vi "Temp_SetTempOrigin.vi"(8 "Z":dbl format="%#_13g", 9 "Y":dbl format="%#_13g", 10 "X":dbl format="%#_13g", 11 "String":string) -> (3 "concatenated string":string)   [LabVIEW 2016]
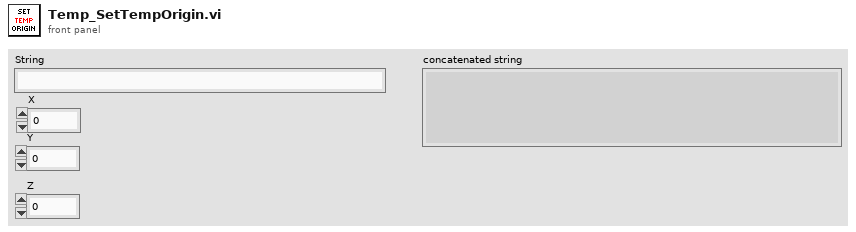
[diagram p1: front panel]
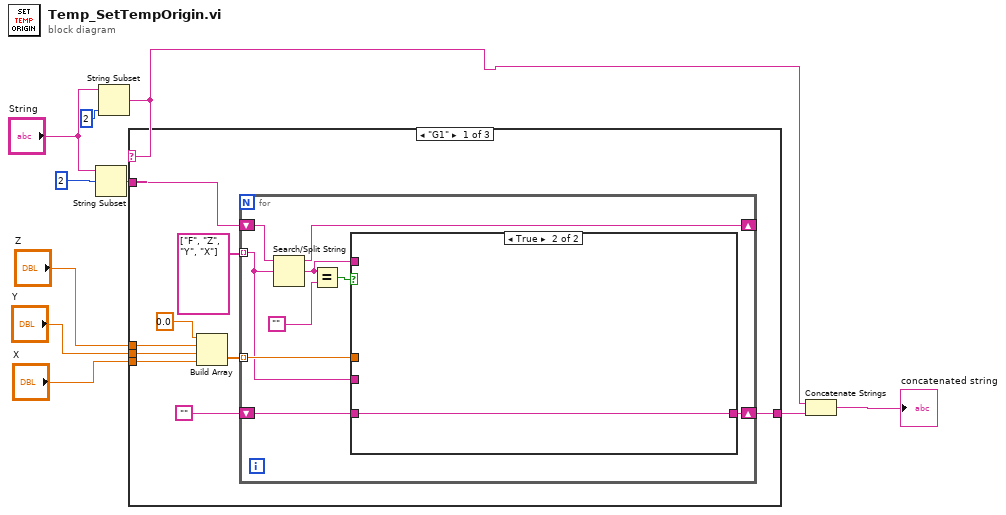
[diagram p0: block diagram]
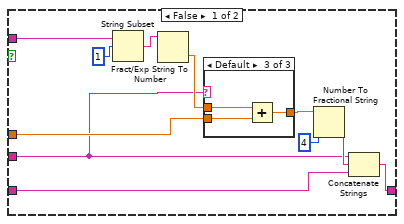
[diagram p2: hidden frame]
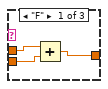
[diagram p3: hidden frame]
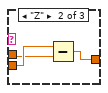
[diagram p4: hidden frame]
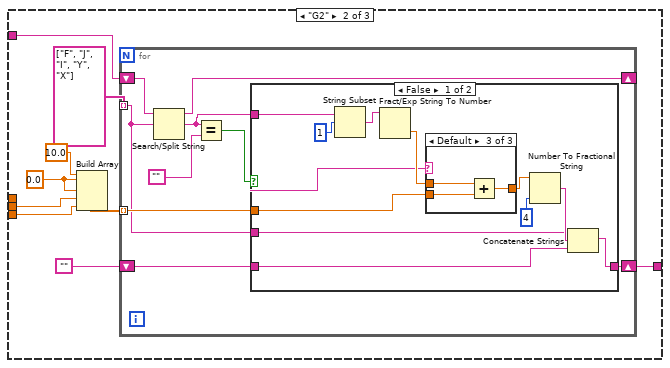
[diagram p5: hidden frame]
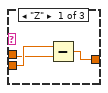
[diagram p6: hidden frame]
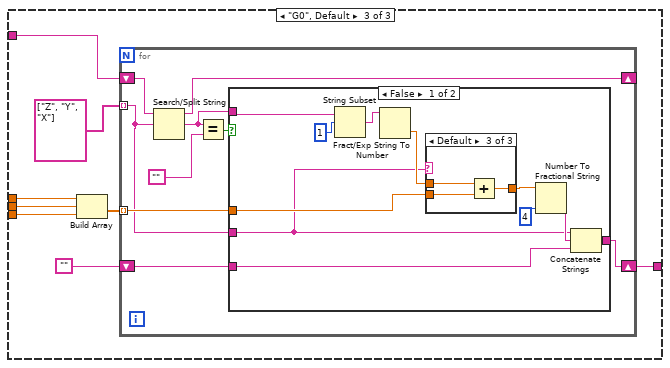
[diagram p9: hidden frame]
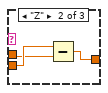
[diagram p11: hidden frame]
diagram:
  n1 = String Subset(string="String", offset (0)=2) -> (substring=w9:string)  [unwired: 1 in]
  n2 = String Subset(string="String", length (rest)=2) -> (substring=w1:string)  [unwired: 1 in]
  n3 = case shown="\"G1\"" w1 {
    tunnel: w9 -> [w18 w57 w94]
    tunnel: "Z" -> [w17 _ w93]
    tunnel: "Y" -> [w16 w51 w92]
    tunnel: "X" -> [w15 w52 w91]
    tunnel: [w11 w54 w88] -> w3
    frame "G1" {
      n4 = Build Array(0.0, w17, w16, w15) -> (w13:dbl[])
      n5 = for {
        tunnel: string[] ["F", "Z", "Y", "X"] -> [w22] mode=indexing
        tunnel: w13 -> [w24] mode=indexing
        shift-right: [w27] -> _
        shift-left: w18 -> [w28]
        shift-right: [w25] -> w11
        shift-left: "" -> [w23]
        n6 = Search/Split String(string=w28, search string/char (-)=w22) -> (substring before match=w27:string, match + rest of string=w20:string)  [unwired: 1 in, 1 out]
        n7 = Equal?(x=w20, y="") -> (x = y?=w21:bool)
        n8 = case shown="True" w21 {
          tunnel: [w34 w49] -> w25
          tunnel: w24 -> [w33 _]
          tunnel: w23 -> [w32 w49]
          tunnel: w22 -> [w31 _]
          tunnel: w20 -> [w29 _]
          frame False {
            n9 = String Subset(string=w29, offset (0)=1) -> (substring=w38:string)  [unwired: 1 in]
            n10 = Fract/Exp String To Number(string=w38) -> (number=w37:dbl)  [unwired: 3 in, 1 out]
            n11 = case shown="Default" w31 {
              tunnel: w37 -> [w41 w43 w48]
              tunnel: [w42 w45 w47] -> w36
              tunnel: w33 -> [w40 w44 w46]
              frame "F" {
                n12 = Add(x=w41, y=w40) -> (x+y=w42:dbl)
              }
              frame "Z" {
                n13 = Subtract(x=w44, y=w43) -> (x-y=w45:dbl)
              }
              frame Default {
                n14 = Add(x=w48, y=w46) -> (x+y=w47:dbl)
              }
            }
            n15 = Number To Fractional String(number=w36, precision (6)=4) -> (F-format string=w35:string)  [unwired: 2 in]
            n16 = Concatenate Strings(w31, w35, w32) -> (w34:string)
          }
          frame True {
          }
        }
      }
    }
    frame "G2" {
      w50 = 0.0
      n17 = Build Array(10.0, w50, w50, w51, w52) -> (w56:dbl[])
      n18 = for {
        tunnel: string[] ["F", "J", "I", "Y", "X"] -> [w61] mode=indexing
        tunnel: w56 -> [w63] mode=indexing
        shift-right: [w66] -> _
        shift-left: w57 -> [w67]
        shift-right: [w64] -> w54
        shift-left: "" -> [w62]
        n19 = Search/Split String(string=w67, search string/char (-)=w61) -> (substring before match=w66:string, match + rest of string=w59:string)  [unwired: 1 in, 1 out]
        n20 = Equal?(x=w59, y="") -> (x = y?=w60:bool)
        n21 = case shown="False" w60 {
          tunnel: [w73 w86] -> w64
          tunnel: w63 -> [w72 _]
          tunnel: w62 -> [w71 w86]
          tunnel: w61 -> [w69 _]
          tunnel: w59 -> [w68 _]
          frame False {
            n22 = String Subset(string=w68, offset (0)=1) -> (substring=w77:string)  [unwired: 1 in]
            n23 = Fract/Exp String To Number(string=w77) -> (number=w76:dbl)  [unwired: 3 in, 1 out]
            n24 = case shown="Default" w69 {
              tunnel: w76 -> [w79 _ w85]
              tunnel: [w81 w82 w84] -> w75
              tunnel: w72 -> [w80 w82 w83]
              frame "Z" {
                n25 = Subtract(x=w80, y=w79) -> (x-y=w81:dbl)
              }
              frame "F" {
              }
              frame Default {
                n26 = Add(x=w85, y=w83) -> (x+y=w84:dbl)
              }
            }
            n27 = Number To Fractional String(number=w75, precision (6)=4) -> (F-format string=w74:string)  [unwired: 2 in]
            n28 = Concatenate Strings(w69, w74, w71) -> (w73:string)
          }
          frame True {
          }
        }
      }
    }
    frame "G0", Default {
      n29 = Build Array(w93, w92, w91) -> (w90:dbl[])
      n30 = for {
        tunnel: string[] ["Z", "Y", "X"] -> [w97] mode=indexing
        tunnel: w90 -> [w99] mode=indexing
        shift-right: [w102] -> _
        shift-left: w94 -> [w103]
        shift-right: [w100] -> w88
        shift-left: "" -> [w98]
        n31 = Search/Split String(string=w103, search string/char (-)=w97) -> (substring before match=w102:string, match + rest of string=w95:string)  [unwired: 1 in, 1 out]
        n32 = Equal?(x=w95, y="") -> (x = y?=w96:bool)
        n33 = case shown="False" w96 {
          tunnel: [w109 w122] -> w100
          tunnel: w99 -> [w108 _]
          tunnel: w98 -> [w107 w122]
          tunnel: w97 -> [w105 _]
          tunnel: w95 -> [w104 _]
          frame False {
            n34 = String Subset(string=w104, offset (0)=1) -> (substring=w113:string)  [unwired: 1 in]
            n35 = Fract/Exp String To Number(string=w113) -> (number=w112:dbl)  [unwired: 3 in, 1 out]
            n36 = case shown="Default" w105 {
              tunnel: w112 -> [_ w116 w121]
              tunnel: [w115 w118 w120] -> w111
              tunnel: w108 -> [w115 w117 w119]
              frame "F" {
              }
              frame "Z" {
                n37 = Subtract(x=w117, y=w116) -> (x-y=w118:dbl)
              }
              frame Default {
                n38 = Add(x=w121, y=w119) -> (x+y=w120:dbl)
              }
            }
            n39 = Number To Fractional String(number=w111, precision (6)=4) -> (F-format string=w110:string)  [unwired: 2 in]
            n40 = Concatenate Strings(w105, w110, w107) -> (w109:string)
          }
          frame True {
          }
        }
      }
    }
  }
  n41 = Concatenate Strings(w1, w3) -> (→"concatenated string":string)
